vi "sv_Flat New Pink Filter Coefficients.vi"(8 "unity gain freq (rad/s)":dbl=1.0 format="%.2g", 10 "fs":dbl=1000.0 format="%.2f", 11 "lower cutoff freq":dbl=0.1) -> (0 "error":i32, 1 "magnitude error (dB)":T2, 2 "filter information":T1, 3 "IIR Filter Cluster":T3 {"Forward Coefficients" format="%.4f"; "Reverse Coefficients" format="%.4f"}, 4 "noise bandwidth":dbl=1.0 format="%.2g")   [LabVIEW 2017]
uses:
  <vilib>/Analysis/3filter.llb/Filter Passband Type.ctl
  <vilib>/Analysis/3filter.llb/Filter Structure Type.ctl
  <vilib>/Analysis/NI_AALBase.lvlib
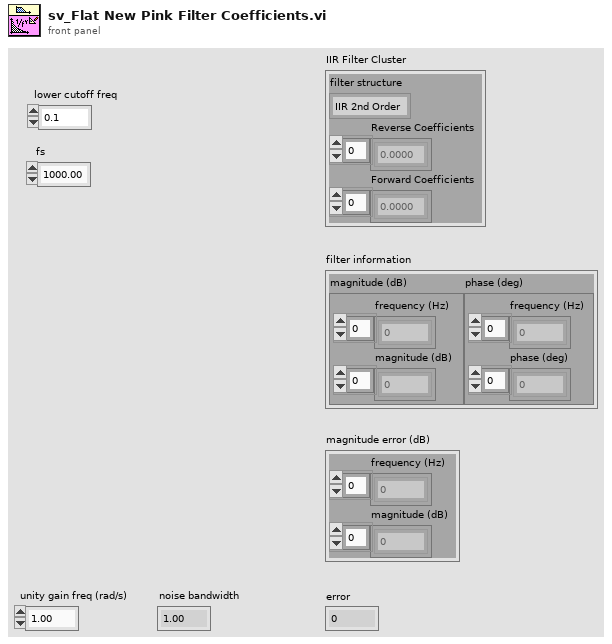
[diagram p1: front panel]
types:
  T1 = cluster{"magnitude (dB)":cluster{"frequency (Hz)":dbl[], "magnitude (dB)":dbl[]}, "phase (deg)":cluster{"frequency (Hz)":dbl[], "phase (deg)":dbl[]}}
  T2 = cluster{"frequency (Hz)":dbl[], "magnitude (dB)":dbl[]}
  T3 = cluster{"filter structure":enum32{"IIR 2nd Order", "IIR 4th Order"}, "Reverse Coefficients":dbl[], "Forward Coefficients":dbl[]}
  T4 = typedef "NI_AALBase.lvlib/Filter Passband Type.ctl" = enum32{"Lowpass", "Highpass", "Bandpass", "Bandstop"}
  T5 = cluster{"Fstart":dbl, "Fstop":dbl, "# points":i32, "type":u16}
  T6 = cluster{"filter structure":enum32{"IIR 2nd Order", "IIR 4th Order"}, "b[i]":dbl[], "b[i]":dbl[]}
  T7 = typedef "NI_AALBase.lvlib/Filter Structure Type.ctl" = u16
  T8 = typedef "sv_Flat Pink Noise Coefficients.ctl" = cluster{"sample rate":dbl, "order":i32, "reference freq":dbl, "coefficients":cluster{"filter structure":enum32{"IIR 2nd Order", "IIR 4th Order"}, "Reverse Coefficients":dbl[], "Forward Coefficients":dbl[]}}
  T9 = cluster{"corrected magnitude (dB)":cluster{"frequency (Hz)":dbl[], "magnitude (dB)":dbl[]}, "Phase (degrees)":cluster{dbl[], dbl[]}}
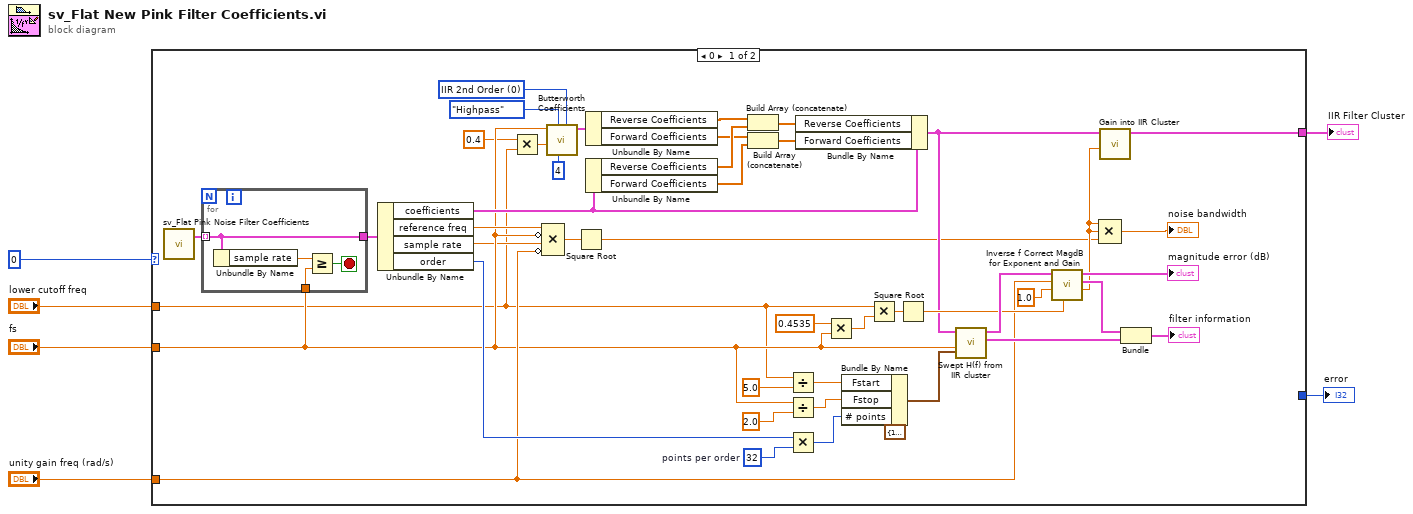
[diagram p0: block diagram]
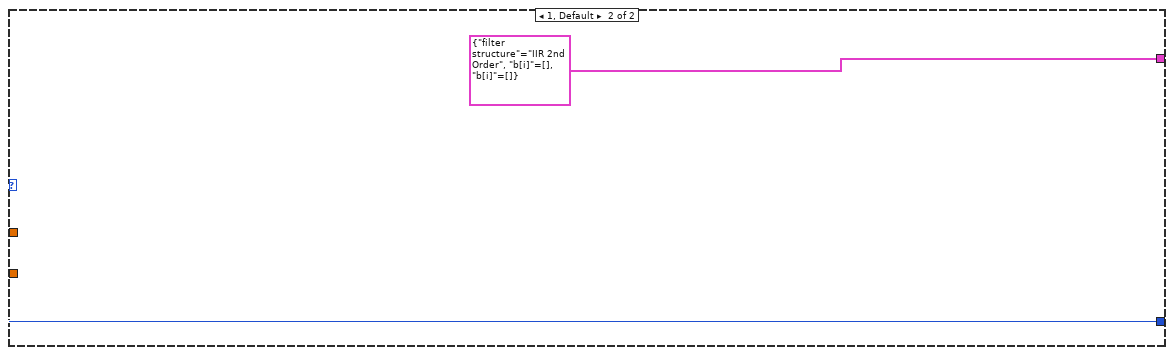
[diagram p2: hidden frame]
diagram:
  n1 = case shown="0" 0 ("error code") {
    selector: 0 ("error code") -> [_ w56]
    tunnel: [w40 T6 {"filter structure"=enum."IIR 2nd Order", "b[i]"=[], "b[i]"=[]}] -> w6
    tunnel: "fs" -> [w11 _]
    tunnel: [_ w56] -> w5
    tunnel: "unity gain freq (rad/s)" -> [w12 _]
    tunnel: "lower cutoff freq" -> [w9 _]
    frame 0 {
      w24 = T7 0 items=["IIR 2nd Order"=0, "IIR 4th Order"=1, "Auto Select"=10] ("filter structure option")
      w49 = 32  # points per order
      n2 = call <vilib>:"sv_Flat Pink Noise Filter Coefficients.vi"() -> ("pink noise coeffs out"=w28:T8[])  [unwired: 3 in]
      n3 = for {
        tunnel: w28 -> [w52] mode=indexing
        tunnel: w11 -> [w54]
        tunnel: [w52] -> w27
        stop <- w53 stop-if-true
        n4 = Unbundle By Name(w52) -> ("sample rate"=w55:dbl)
        n5 = Greater Or Equal?(x=w55, y=w54) -> (x >= y?=w53:bool)
      }
      n6 = Unbundle By Name(w27) -> ("coefficients"=w13:T3, "reference freq"=w31:dbl, "sample rate"=w10:dbl, "order"=w29:i32)
      n7 = Multiply(x=0.4, y=w9) -> (x*y=w8:dbl)
      n8 = Compound Arithmetic op=MULTIPLY(w31, invert w11, w10, invert w12) -> (w30:dbl)
      n9 = call <vilib>:"Butterworth Coefficients.vi"("filter structure option"=w24, "order"=4, "filter type"=Filter_Passband_Type."Highpass", "low cutoff freq: fl"=w8, "sampling freq: fs"=w11) -> ("IIR Filter Cluster"=w19:T3)  [unwired: 5 in, 1 out]
      n10 = Square Root(x=w30) -> (sqrt(x)=w14:dbl)
      n11 = Unbundle By Name(w19) -> ("Reverse Coefficients"=w23:dbl[], "Forward Coefficients"=w21:dbl[])
      n12 = Unbundle By Name(w13) -> ("Reverse Coefficients"=w22:dbl[], "Forward Coefficients"=w20:dbl[])
      n13 = Build Array (concatenate)(w23, w22) -> (w18:dbl[])
      n14 = Build Array (concatenate)(w21, w20) -> (w17:dbl[])
      n15 = Divide(x=w9, y=5.0) -> (x/y=w45:dbl)
      n16 = Divide(x=w11, y=2.0) -> (x/y=w44:dbl)
      n17 = Multiply(x=w29, y=w49) -> (x*y=w48:i32)
      n18 = Bundle By Name(cluster=w13, "Reverse Coefficients"=w18, "Forward Coefficients"=w17) -> (w16:T3)
      n19 = Multiply(x=0.4535, y=w11) -> (x*y=w34:dbl)
      n20 = Bundle By Name(cluster=T5 {"Fstart"=1e-06, "Fstop"=0.4, "# points"=100, "type"=1} ("Sweep specs"), "Fstart"=w45, "Fstop"=w44, "# points"=w48) -> (w46:T5)
      n21 = Multiply(x=w9, y=w34) -> (x*y=w43:dbl)
      n22 = Square Root(x=w43) -> (sqrt(x)=w42:dbl)
      n23 = call <vilib>:"Swept H(f) from IIR cluster.vi"("Sweep specs"=w46, "Fs"=w11, "IIR Filter Cluster"=w16) -> ("Phase (degrees)"=w50:cluster{dbl[], dbl[]}, "Magnitude (dB)"=w47:cluster{dbl[], dbl[]})  [unwired: 7 in]
      n24 = call <vilib>:"Inverse f Correct MagdB for Exponent and Gain.vi"("alignment frequency (Hz)"=w42, "exponent"=1.0, "unity gain freq (rd/s)"=w12, "magnitude (dB)"=w47) -> ("gain to apply"=w15:dbl, "corrected magnitude (dB)"=w41:T2, "magnitude error (dB)"=→"magnitude error (dB)":T2)  [unwired: 5 in]
      n25 = Compound Arithmetic op=MULTIPLY(w15, w15, w14) -> (→"noise bandwidth":dbl)
      n26 = call <vilib>:"Gain into IIR Cluster.vi"("gain"=w15, "IIR Filter Cluster in"=w16) -> ("IIR Filter Cluster out"=w40:T3)  [unwired: 9 in]
      n27 = Bundle("corrected magnitude (dB)"=w41, "Phase (degrees)"=w50) -> (→"filter information":T9)  [unwired: 1 in]
    }
    frame 1, Default {
    }
  }
  "error" <- w5
  "IIR Filter Cluster" <- w6
